vi "AlliGator Load HDF5 FLI Header File Information v0.6.vi"(8 "error in (no error)":errorcluster, 10 "HDF5 FLI File Loading Information":T1, 11 "ref in":T2 format="%.0x") -> (0 "error out":errorcluster, 1 "File Information String":string, 2 "HDF5 FLI File Loading Information out":T1, 3 "ref out":T2 format="%.0x")   [LabVIEW 2021, in "AlliGator HDF5.lvlib"]
doc: "Loads HDF5 FLI dataset file information (v0.6)."
uses:
  AlliGator HDF5.lvlib
  <vilib>/addons/h5labview2/base/hid_t.ctl
  AlliGator HDF5 FLI File Loading Information v0.6.ctl
  <vilib>/addons/h5labview2/base/lib_path.vi
  <vilib>/addons/h5labview2/base/H5Equery.vi
  <vilib>/addons/h5labview2/dataset/H5Dread.llb/H5Dread.xnode
  Strings/Strings.lvlib
panel:
  out "Header error":errorcluster
  # "see the AlliGator License on the block diagram (Ctrl+E or Window:Show Block Diagram)"
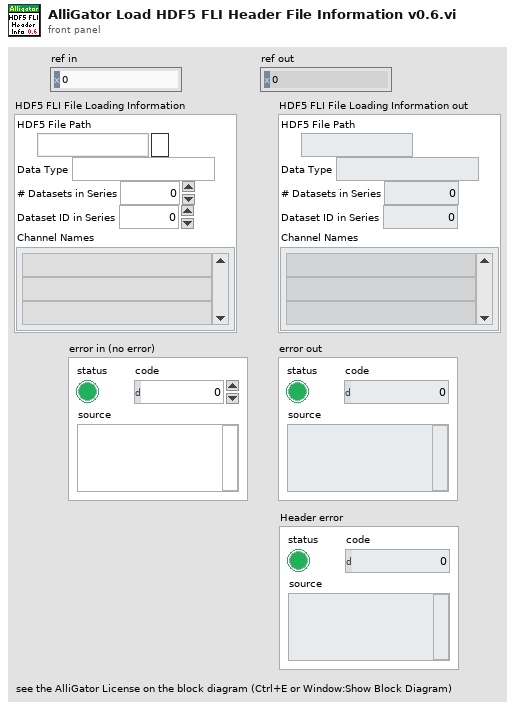
[diagram p1: front panel]
types:
  T1 = typedef "AlliGator HDF5.lvlib/AlliGator HDF5 FLI File Loading Information v0.6.ctl" = cluster{"HDF5 File Path":path, "Data Type":string, "# Datasets in Series":i32, "Dataset ID in Series":i32, "Channel Names":string[]}
  T2 = typedef "hid_t.ctl" = i64
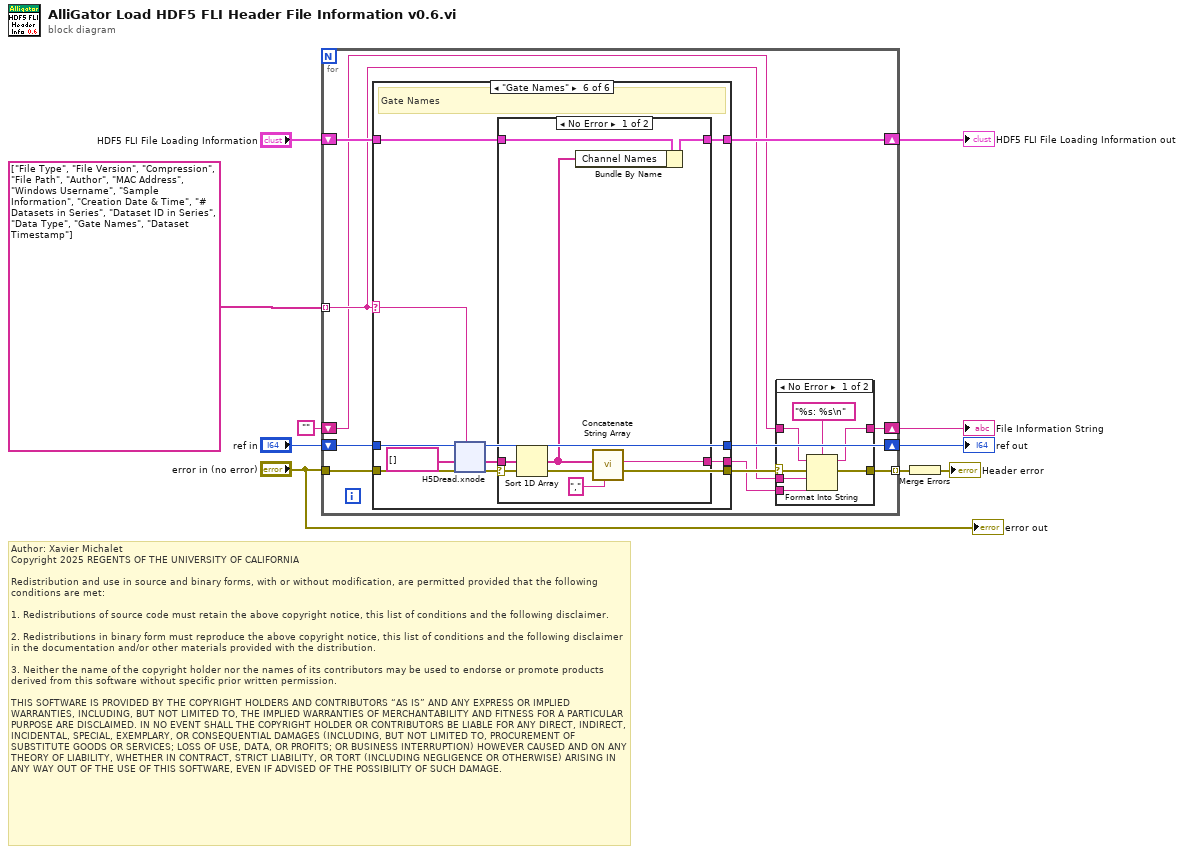
[diagram p0: block diagram]
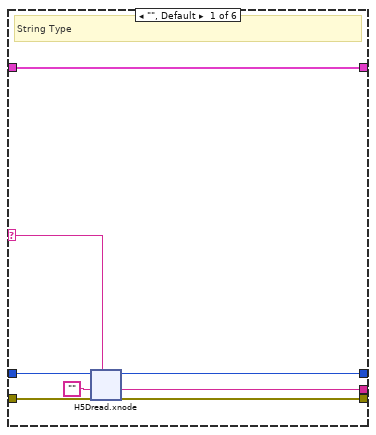
[diagram p3: hidden frame]
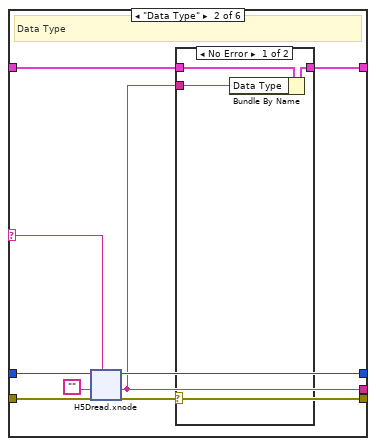
[diagram p4: hidden frame]
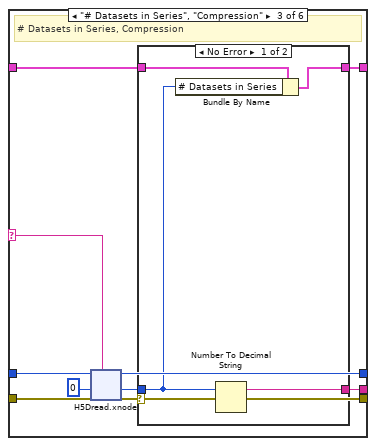
[diagram p6: hidden frame]
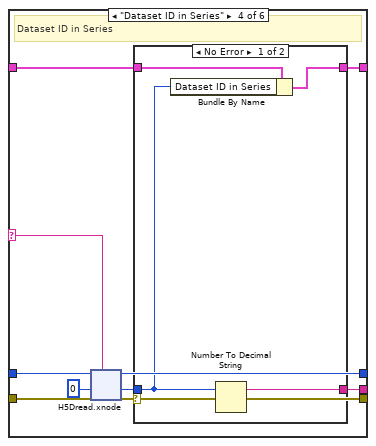
[diagram p8: hidden frame]
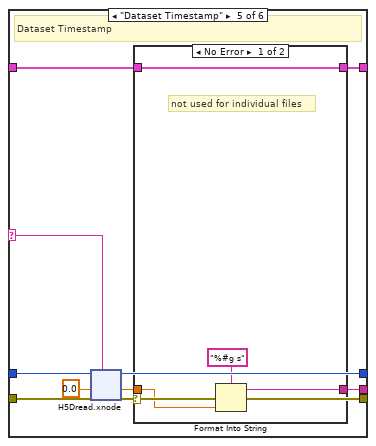
[diagram p10: hidden frame]
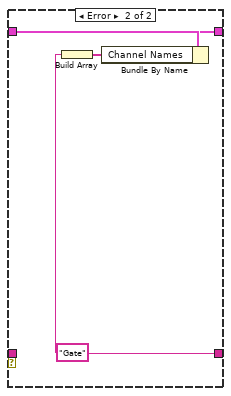
[diagram p12: hidden frame]
diagram:
  # "Author: Xavier Michalet\nCopyright 2025 REGENTS OF THE UNIVERSITY OF CALIFORNIA\n\nRedistribution and use in source and binary forms, with or without modification, are permitted provided that the following conditions are met:\n\n1. Redistributions of source code must retain the above copyright notice, this list of conditions and the following disclaimer.\n\n2. Redistributions in binary form must reproduce the above copyright notice, this list of conditions and the following disclaimer in the documentation and/or other materials provided with the distribution.\n\n3. Neither the name of the copyright holder nor the names of its contributors may be used to endorse or promote products derived from this software without specific prior written permission.\n\nTHIS SOFTWARE IS PROVIDED BY THE COPYRIGHT HOLDERS AND CONTRIBUTORS “AS IS” AND ANY EXPRESS OR IMPLIED WARRANTIES, INCLUDING, BUT NOT LIMITED TO, THE IMPLIED WARRANTIES OF MERCHANTABILITY AND FITNESS FOR A PARTICULAR PURPOSE ARE DISCLAIMED. IN NO EVENT SHALL THE COPYRIGHT HOLDER OR CONTRIBUTORS BE LIABLE FOR ANY DIRECT, INDIRECT, INCIDENTAL, SPECIAL, EXEMPLARY, OR CONSEQUENTIAL DAMAGES (INCLUDING, BUT NOT LIMITED TO, PROCUREMENT OF SUBSTITUTE GOODS OR SERVICES; LOSS OF USE, DATA, OR PROFITS; OR BUSINESS INTERRUPTION) HOWEVER CAUSED AND ON ANY THEORY OF LIABILITY, WHETHER IN CONTRACT, STRICT LIABILITY, OR TORT (INCLUDING NEGLIGENCE OR OTHERWISE) ARISING IN ANY WAY OUT OF THE USE OF THIS SOFTWARE, EVEN IF ADVISED OF THE POSSIBILITY OF SUCH DAMAGE."
  n1 = for {
    shift-right: [w19] -> w7
    shift-left: "ref in" -> [w21]
    tunnel: string[] ["File Type", "File Version", "Compression", "File Path", "Author", "MAC Address", "Windows Username", "Sample Information", "Creation Date & Time", "# Datasets in Series", "Dataset ID in Series", "Data Type", "Gate Names", "Dataset Timestamp"] ("dataset name") -> [w12] mode=indexing
    shift-right: [w15] -> w10
    shift-left: "" -> [w11]
    shift-right: [w13] -> w4
    shift-left: "HDF5 FLI File Loading Information" -> [w14]
    tunnel: "error in (no error)" -> [w20]
    tunnel: [w17] -> w3 mode=indexing
    n2 = case shown="\"Gate Names\"" w12 {
      selector: w12 -> [w35 w59 w88 w118 w148 w179]
      tunnel: w21 -> [w38 w62 w91 w121 w151 w182]
      tunnel: w20 -> [w37 w61 w90 w120 w150 w181]
      tunnel: [w36 w60 w89 w119 w149 w180] -> w19
      tunnel: [w31 w54 w82 w112 w142 w174] -> w18
      tunnel: [w34 w55 w83 w113 w143 w175] -> w16
      tunnel: w14 -> [w32 w57 w87 w117 w147 w178]
      tunnel: [w32 w56 w86 w116 w146 w177] -> w13
      frame "", Default {
        # "String Type"
        n3 = xnode "H5Dread.xnode"("dataset name (this)"=w35, "error in (no error)"=w37, "default"="", "ref in"=w38) -> ("error out"=w31:errorcluster, "data"=w34:string, "ref out"=w36:T2)  [unwired: 2 in, 1 out]
      }
      frame "Data Type" {
        # "Data Type"
        n4 = xnode "H5Dread.xnode"("dataset name (this)"=w59, "error in (no error)"=w61, "default"="", "ref in"=w62) -> ("error out"=w54:errorcluster, "data"=w55:string, "ref out"=w60:T2)  [unwired: 2 in, 1 out]
        n5 = case shown="No Error" w54 {
          tunnel: w57 -> [w65 w66]
          tunnel: [w64 w66] -> w56
          tunnel: w55 -> [w63 _]
          frame No Error {
            n6 = Bundle By Name(cluster=w65, "Data Type"=w63) -> (w64:T1)
          }
          frame Error {
          }
        }
      }
      frame "# Datasets in Series", "Compression" {
        # "# Datasets in Series, Compression"
        n7 = xnode "H5Dread.xnode"("dataset name (this)"=w88, "error in (no error)"=w90, "default"=0, "ref in"=w91) -> ("error out"=w82:errorcluster, "data"=w85:i32, "ref out"=w89:T2)  [unwired: 2 in, 1 out]
        n8 = case shown="No Error" w82 {
          tunnel: w87 -> [w95 w96]
          tunnel: [w94 w96] -> w86
          tunnel: w85 -> [w93 _]
          tunnel: [w92 _] -> w83
          frame No Error {
            n9 = Bundle By Name(cluster=w95, "# Datasets in Series"=w93) -> (w94:T1)
            n10 = Number To Decimal String(number=w93) -> (decimal integer string=w92:string)  [unwired: 1 in]
          }
          frame Error {
          }
        }
      }
      frame "Dataset ID in Series" {
        # "Dataset ID in Series"
        n11 = xnode "H5Dread.xnode"("dataset name (this)"=w118, "error in (no error)"=w120, "default"=0, "ref in"=w121) -> ("error out"=w112:errorcluster, "data"=w115:i32, "ref out"=w119:T2)  [unwired: 2 in, 1 out]
        n12 = case shown="No Error" w112 {
          tunnel: w117 -> [w125 w126]
          tunnel: [w124 w126] -> w116
          tunnel: w115 -> [w123 _]
          tunnel: [w122 _] -> w113
          frame No Error {
            n13 = Bundle By Name(cluster=w125, "Dataset ID in Series"=w123) -> (w124:T1)
            n14 = Number To Decimal String(number=w123) -> (decimal integer string=w122:string)  [unwired: 1 in]
          }
          frame Error {
          }
        }
      }
      frame "Dataset Timestamp" {
        # "Dataset Timestamp"
        n15 = xnode "H5Dread.xnode"("dataset name (this)"=w148, "error in (no error)"=w150, "default"=0.0, "ref in"=w151) -> ("error out"=w142:errorcluster, "data"=w145:dbl, "ref out"=w149:T2)  [unwired: 2 in, 1 out]
        n16 = case shown="No Error" w142 {
          selector: w142 -> [w155 _]
          tunnel: w147 -> [w152 w157]
          tunnel: [w152 w157] -> w146
          tunnel: w145 -> [w156 _]
          tunnel: [w153 _] -> w143
          frame No Error {
            # "not used for individual files"
            n17 = Format Into String(format string="%#g s", error in=w155, w156) -> (resulting string=w153:string)  [unwired: 1 in, 1 out]
          }
          frame Error {
          }
        }
      }
      frame "Gate Names" {
        # "Gate Names"
        n18 = xnode "H5Dread.xnode"("dataset name (this)"=w179, "error in (no error)"=w181, "default"=string[] [], "ref in"=w182) -> ("error out"=w174:errorcluster, "data"=w176:string[], "ref out"=w180:T2)  [unwired: 2 in, 1 out]
        n19 = case shown="No Error" w174 {
          tunnel: w178 -> [w188 w192]
          tunnel: [w187 w191] -> w177
          tunnel: w176 -> [w183 _]
          tunnel: [w185 w190] -> w175
          frame No Error {
            n20 = Sort 1D Array(array=w183) -> (sorted array=w184:string[])
            n21 = Bundle By Name(cluster=w188, "Channel Names"=w184) -> (w187:T1)
            n22 = call "Concatenate String Array.vi"("Separator (TAB)"=",", "String Array"=w184) -> ("Formatted String"=w185:string)  [unwired: 9 in]
          }
          frame Error {
            w190 = "Gate" ("String")
            n23 = Build Array(w190) -> (w189:string[])
            n24 = Bundle By Name(cluster=w192, "Channel Names"=w189) -> (w191:T1)
          }
        }
      }
    }
    n25 = case shown="No Error" w18 {
      selector: w18 -> [w28 w29]
      tunnel: [w27 w29] -> w17
      tunnel: w12 -> [w26 _]
      tunnel: w16 -> [w25 _]
      tunnel: [w24 w30] -> w15
      tunnel: w11 -> [w23 w30]
      frame No Error {
        n26 = Format Into String(format string="%s: %s\n", initial string=w23, error in=w28, w26, w25) -> (resulting string=w24:string, error out=w27:errorcluster)
      }
      frame Error {
      }
    }
  }
  "File Information String" <- w10
  "ref out" <- w7
  "HDF5 FLI File Loading Information out" <- w4
  n27 = Merge Errors(w3) -> (→"Header error":errorcluster)
  "error out" <- "error in (no error)"
